vi "TCP command response.vi"(11 "Command String In":string) -> (0 "Correct Ending":bool, 3 "TCP send this string":string)   [LabVIEW 2014]
uses:
  <vilib>/regexp/Match Regular Expression.xnode
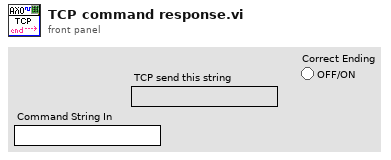
[diagram p1: front panel]
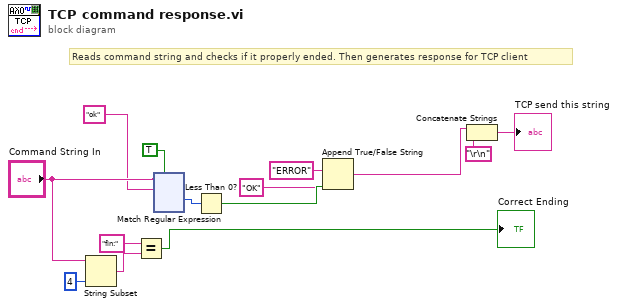
[diagram p0: block diagram]
diagram:
  # "Reads command string and checks if it properly ended. Then generates response for TCP client"
  n1 = String Subset(string="Command String In", length (rest)=4 ("length (rest)")) -> (substring=w11:string)  [unwired: 1 in]
  n2 = Equal?(x="fin:", y=w11) -> (x = y?=→"Correct Ending":bool)
  n3 = xnode "Match Regular Expression"("input string"="Command String In", "regular expression"="ok", "ignore case? (F)"=TRUE) -> ("offset past match"=w5:i32)  [unwired: 3 in, 4 out]
  n4 = Less Than 0?(x=w5) -> (x < 0?=w4:bool)
  n5 = Append True/False String(1:w4, 2:"OK" ("false string"), 3:"ERROR" ("true string")) -> (0:w1:string)  [unwired: 1 in]
  n6 = Concatenate Strings(w1, "\r\n") -> (→"TCP send this string":string)
